vi "Device_without_barcode.vi"() -> ()   [LabVIEW 2016]
uses:
  Global_Valves.vi
  <vilib>/Utility/file.llb/Read Delimited Spreadsheet (I64).vi
panel:
  out "Plugs produced":dbl
  out "Elapsed time (min)":dbl
  out "Start time":timestamp
  out "Number of plugs":i64
  out "Duration of experiment (min)":dbl
  out "Horizontal Graduated Bar":u8(slide) max=66 scale=0.0..66.0
  out "Produced replicas":i32
  out "Inlets Flow On":bool[](array[boolean])
  out "Current condition":i32
  out "Current experiment iteration":i32
  in  "Abort":bool
  in  "Time-out Time":i32
  in  "Port":u16
  in  "Address":string
  out "Time Stamp":timestamp
  in  "Run experiment Button":bool
  out "Experiment running Led":bool
  in  "Experiment File":path
  out "Conditions with replica numbers":i64[][](array[numeric])
  out "Conditions array":i64[][](array[numeric])
  out "Replica numbers":i64[][](array[numeric])
  in  "Iterations of experiment":i32
  in  "Time of depressurization (ms)":u32
  in  "Time of pressurization (ms)":u32
  in  "Time of barcoding (ms)":u32
  in  "Inlet 9":bool
  in  "Inlet 10":bool
  in  "Inlet 11":bool
  in  "Inlet 12":bool
  in  "Inlet 13":bool
  in  "Inlet 14":bool
  in  "Inlet 15":bool
  in  "Inlet 16":bool
  out "Rows":i32
  out "Columns":i32
  in  "Pressurize all channels":bool
  in  "Depressurize all channels":bool
  in  "16":bool
  in  "15":bool
  in  "14":bool
  in  "13":bool
  in  "12":bool
  in  "11":bool
  in  "10":bool
  in  "9":bool
  in  "Stop button":bool
  # "Control \nChannels Manual Pressurization"
  # "Automatic Experiment"
  # "9"
  # "10"
  # "11"
  # "12"
  # "Barcode inlets"
  # "13"
  # "14"
  # "15"
  # "The Barcode Inlets buttons are not controlling anything\nYou can run the experiment without providing the barcode inlets.\n\nThe \"time of barcoding\" will be the time in between the different conditions, during which time all of the control channels are going to be pressurized and only oil will flow."
  # "16"
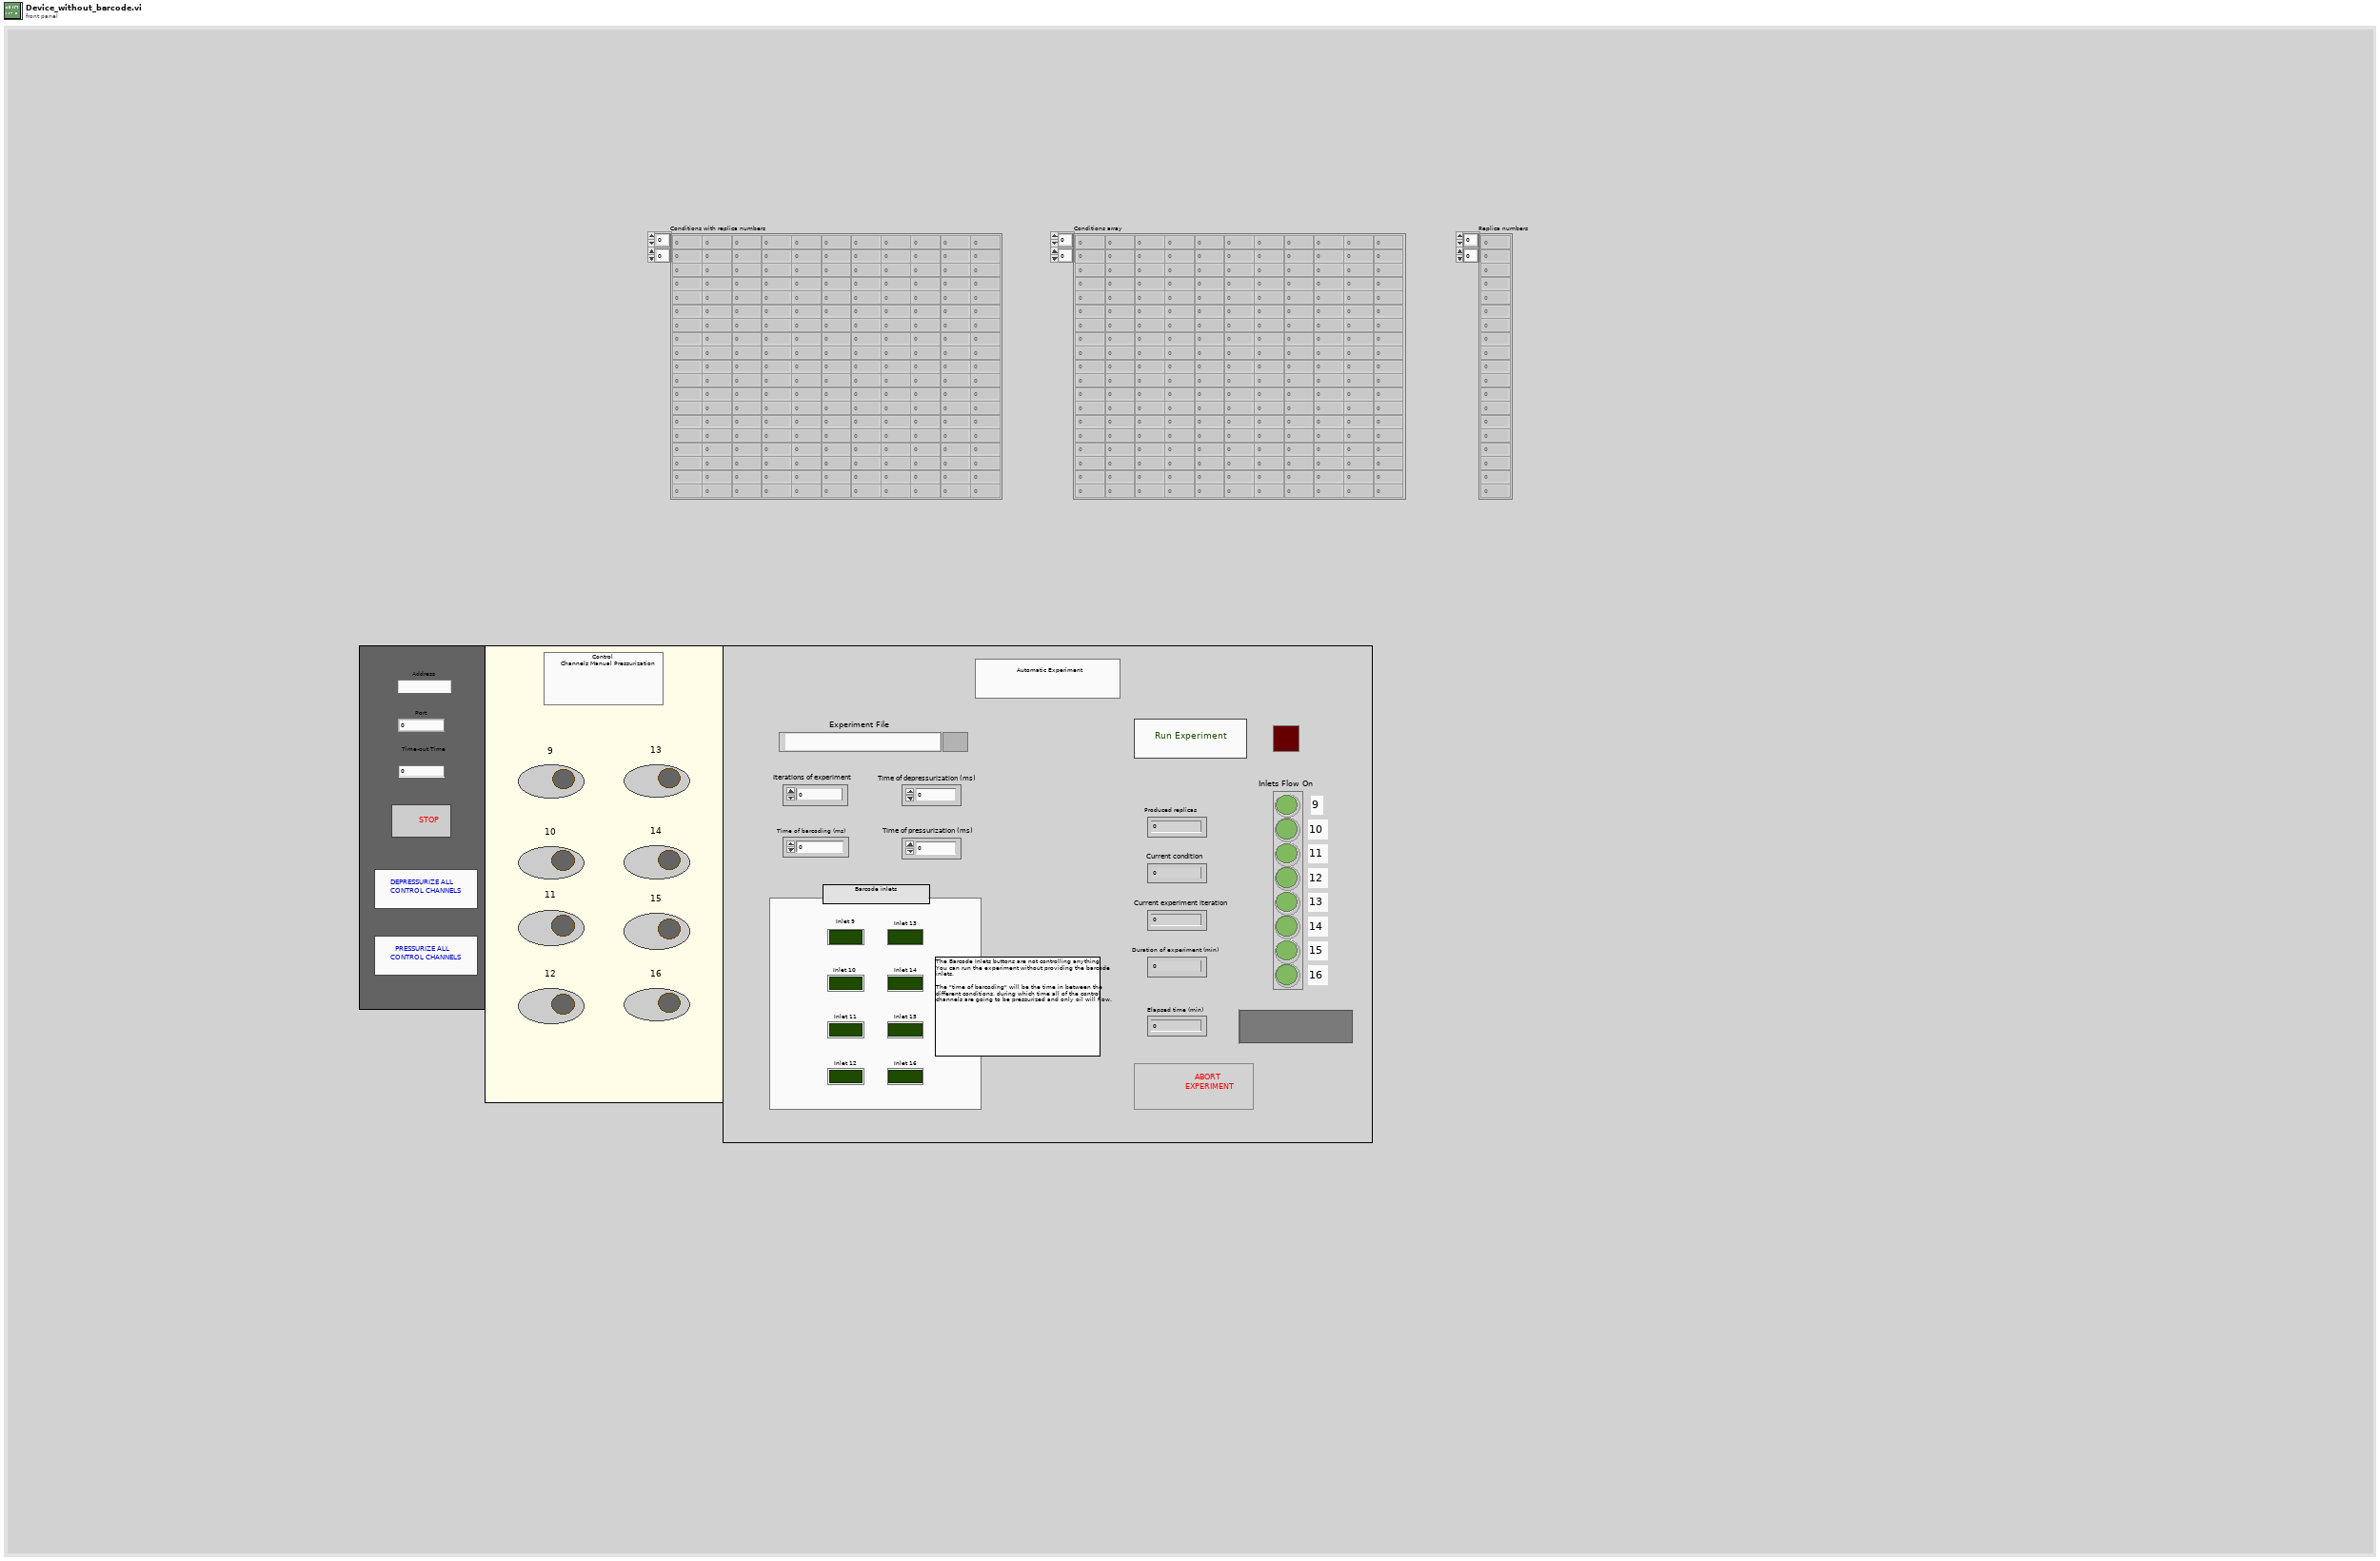
[diagram p1: front panel]
types:
  T1 = enum16{"Start", "Plug replicas production", "Barcoding", "Stop"}
  T2 = enum16{"Start", "Production of plug", "Close inlets", "Stop"}
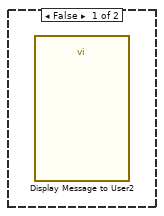
[diagram p2: hidden frame]
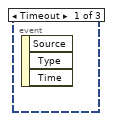
[diagram p4: hidden frame]
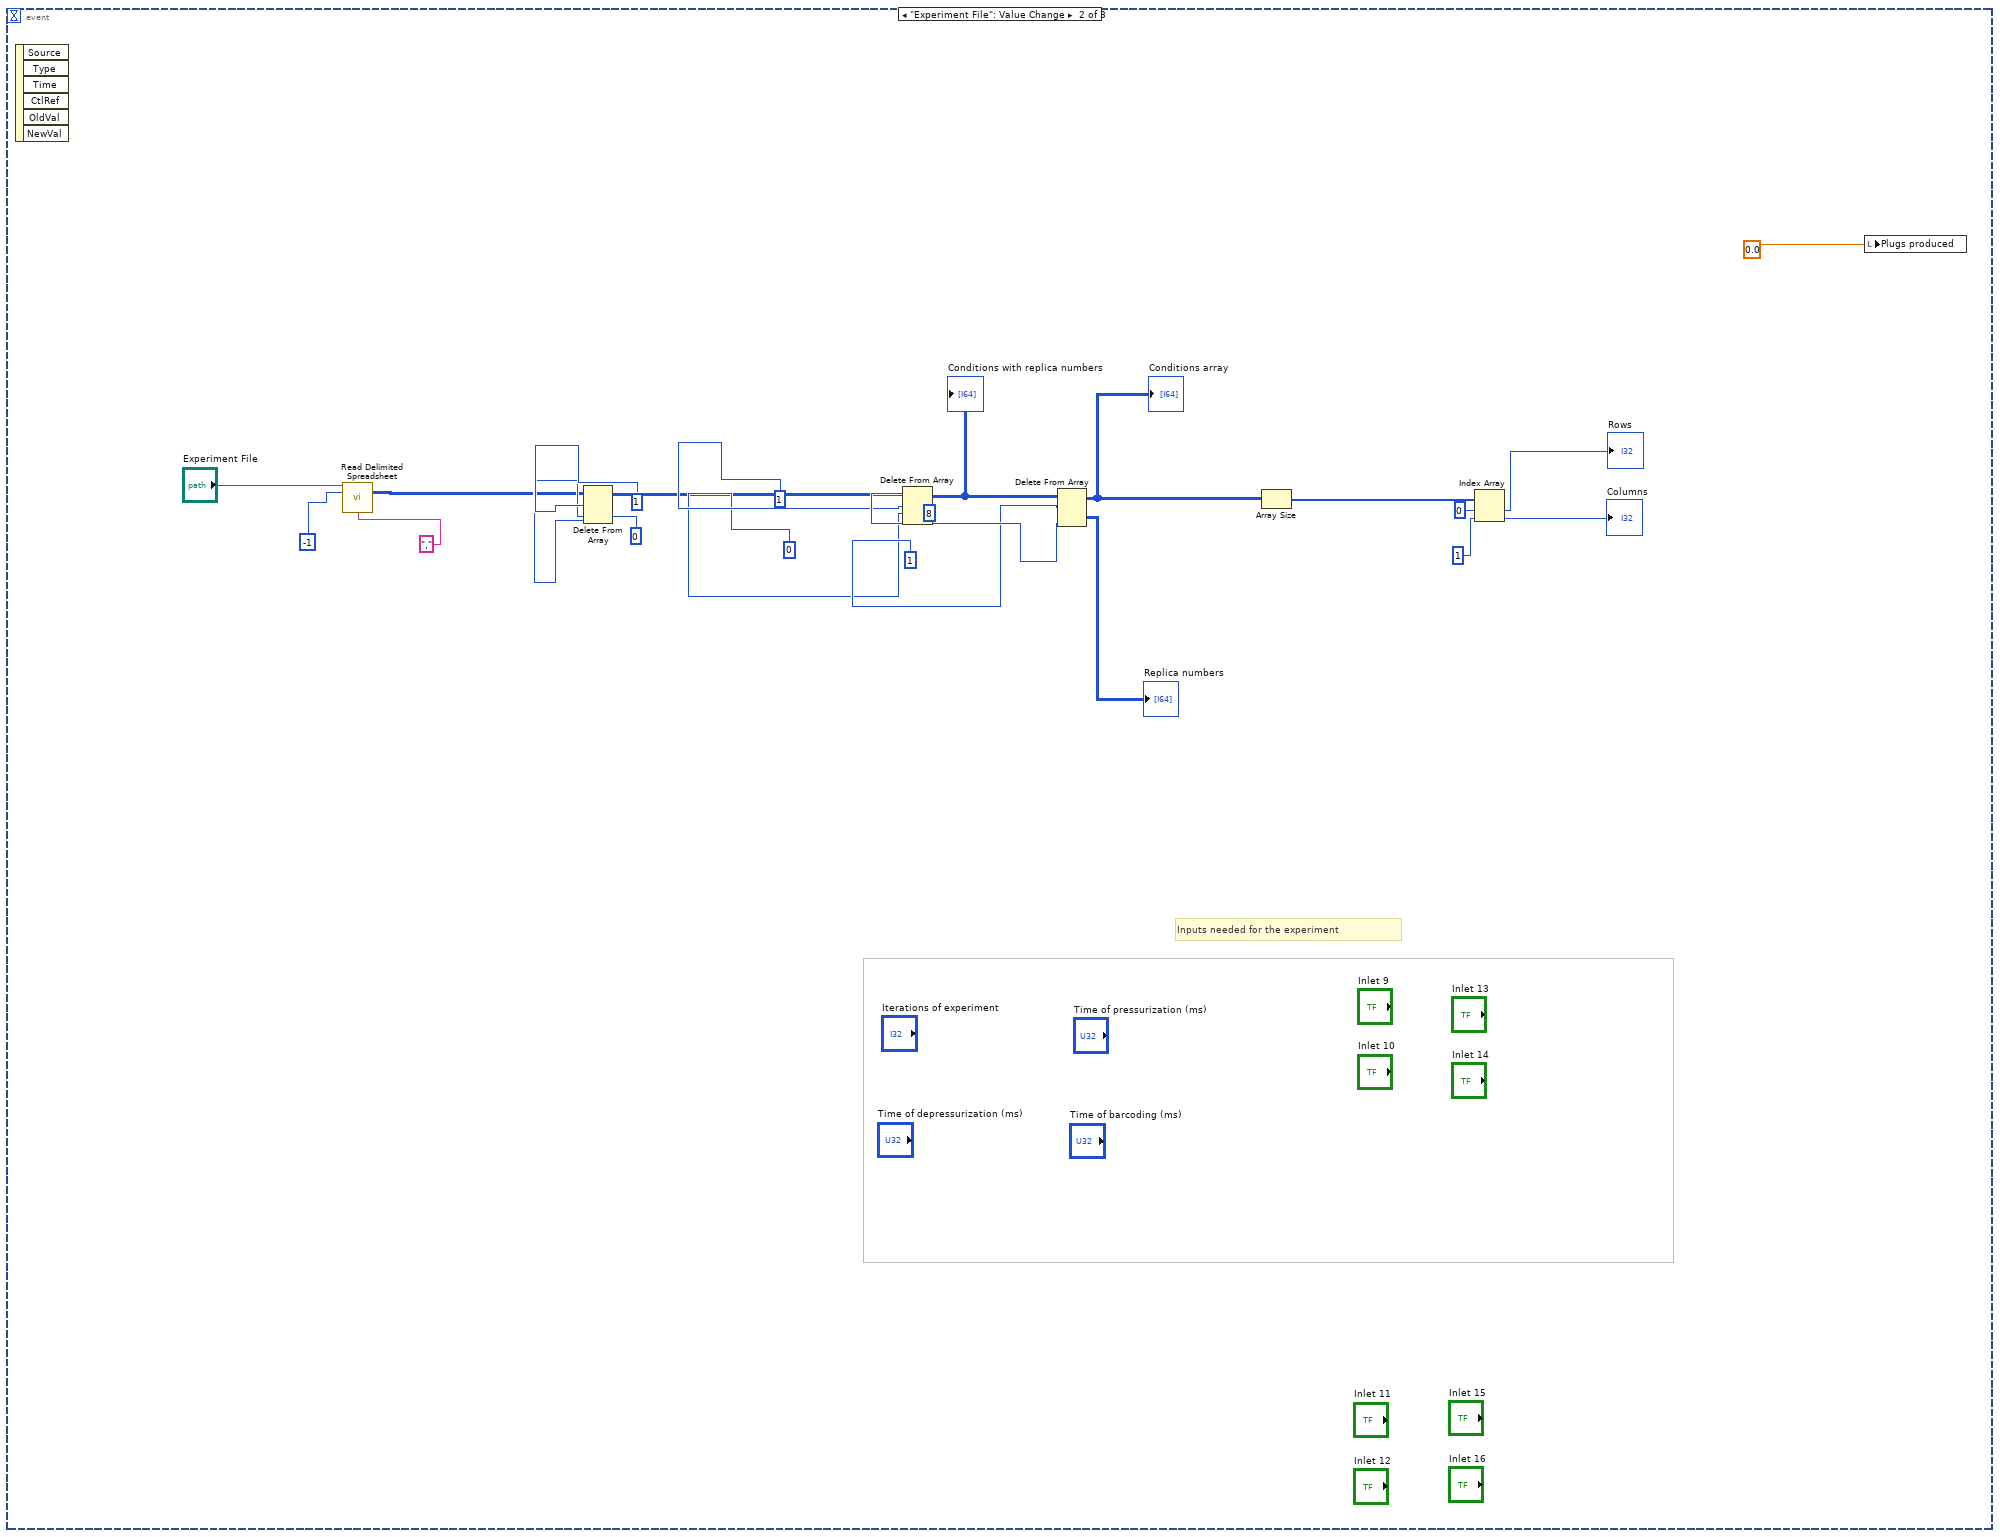
[diagram p5: hidden frame]
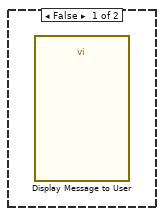
[diagram p6: hidden frame]
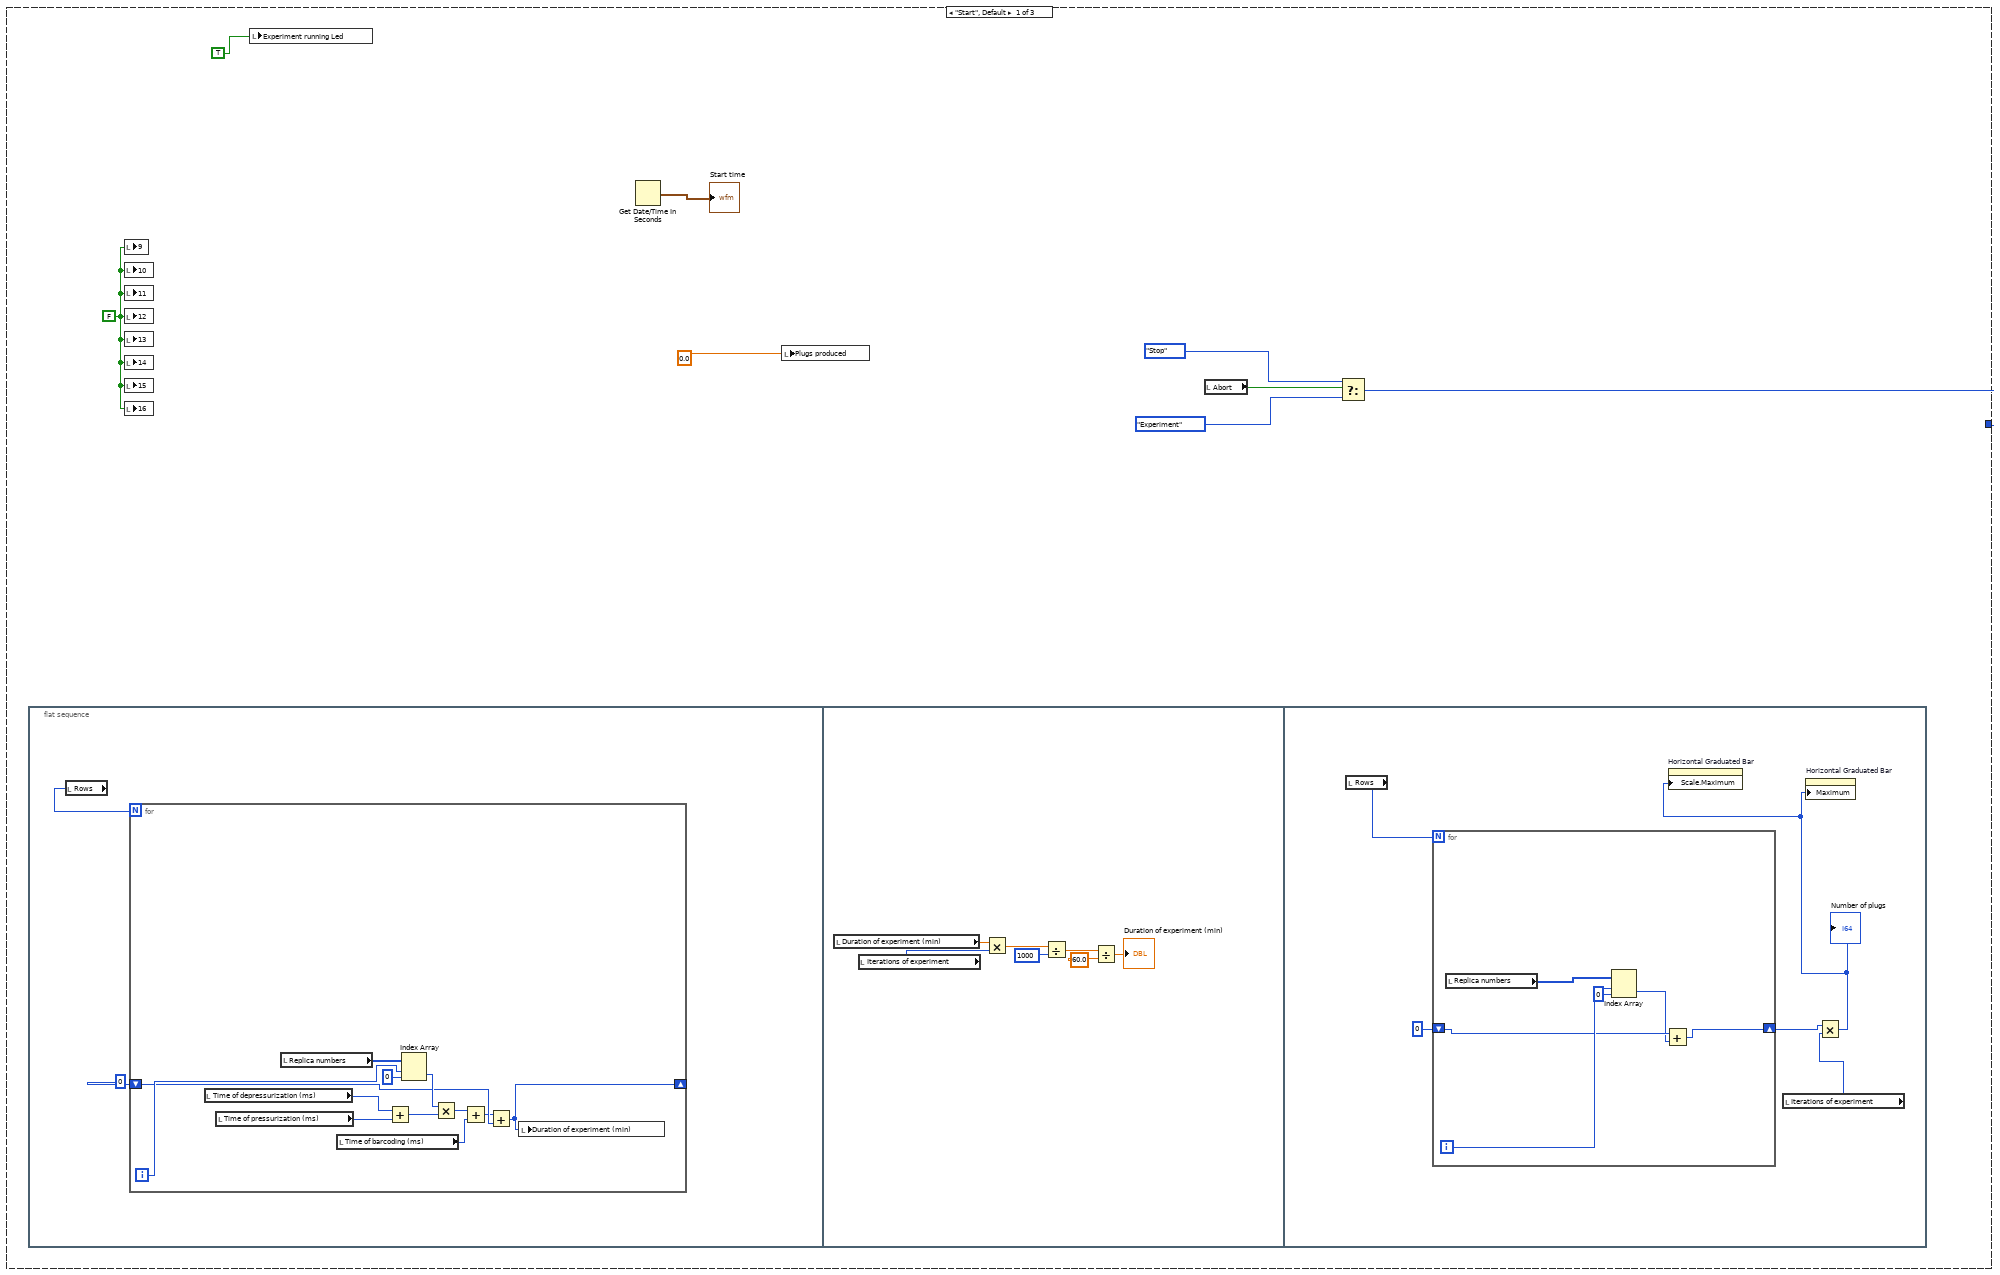
[diagram p7: hidden frame]
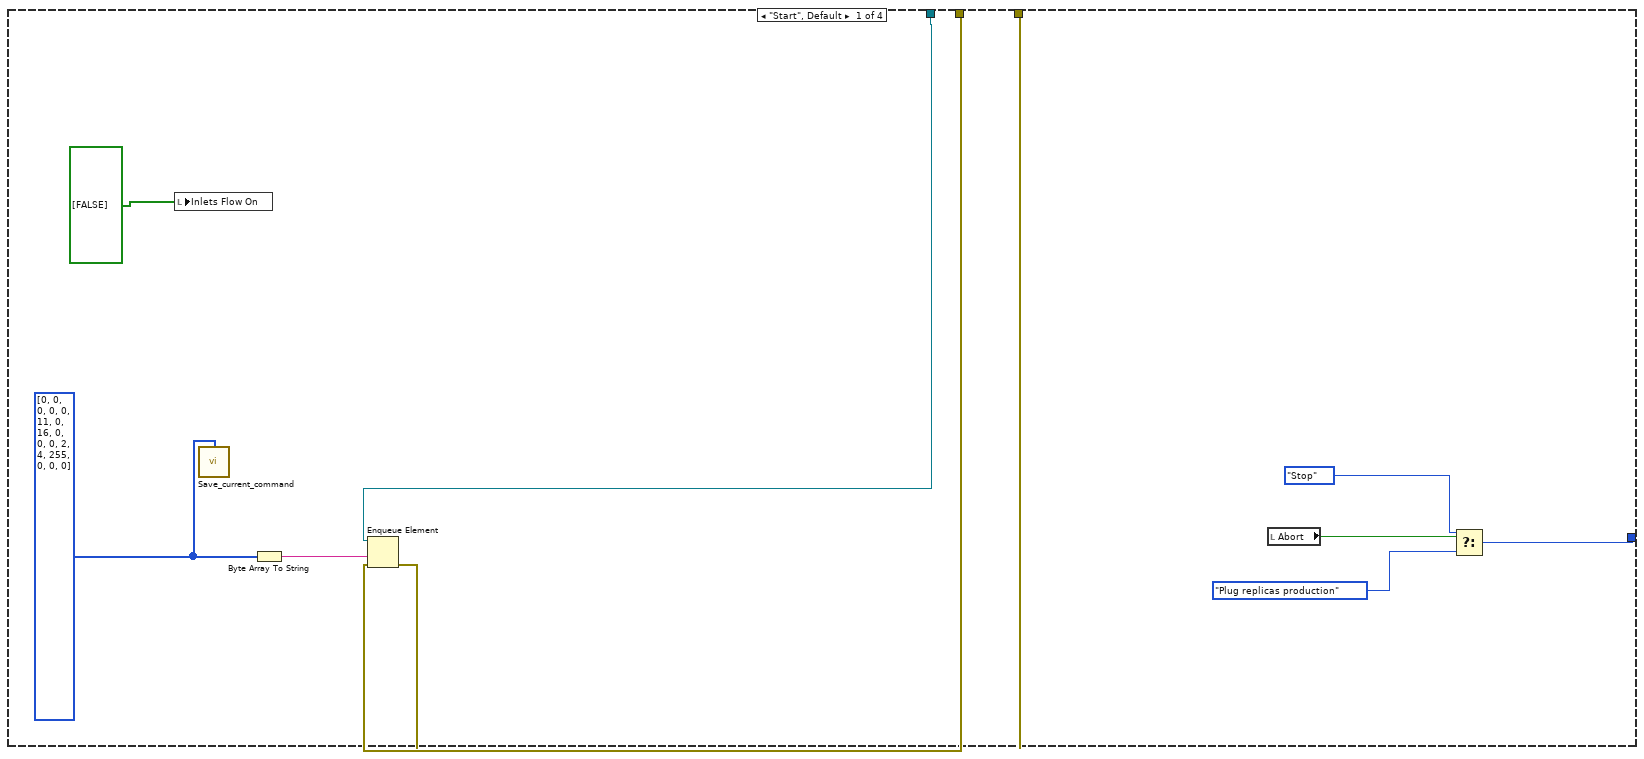
[diagram p8: hidden frame]
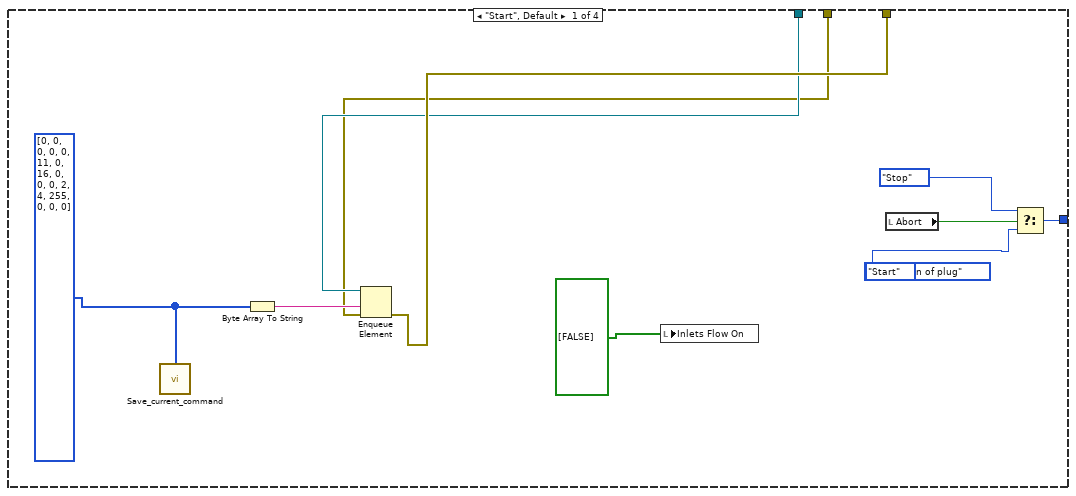
[diagram p9: hidden frame]
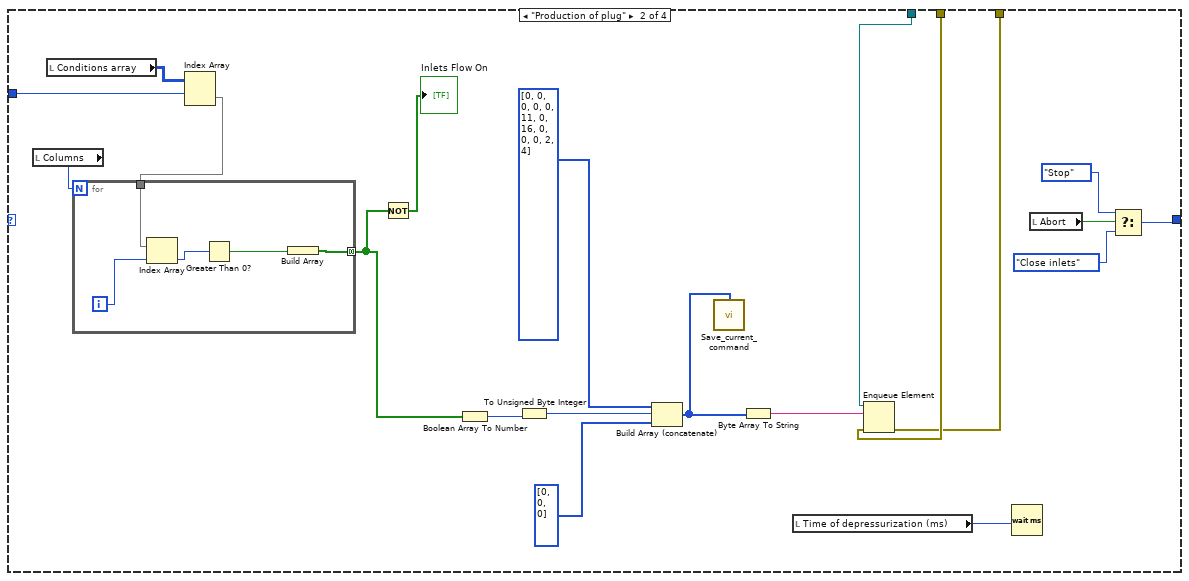
[diagram p10: hidden frame]
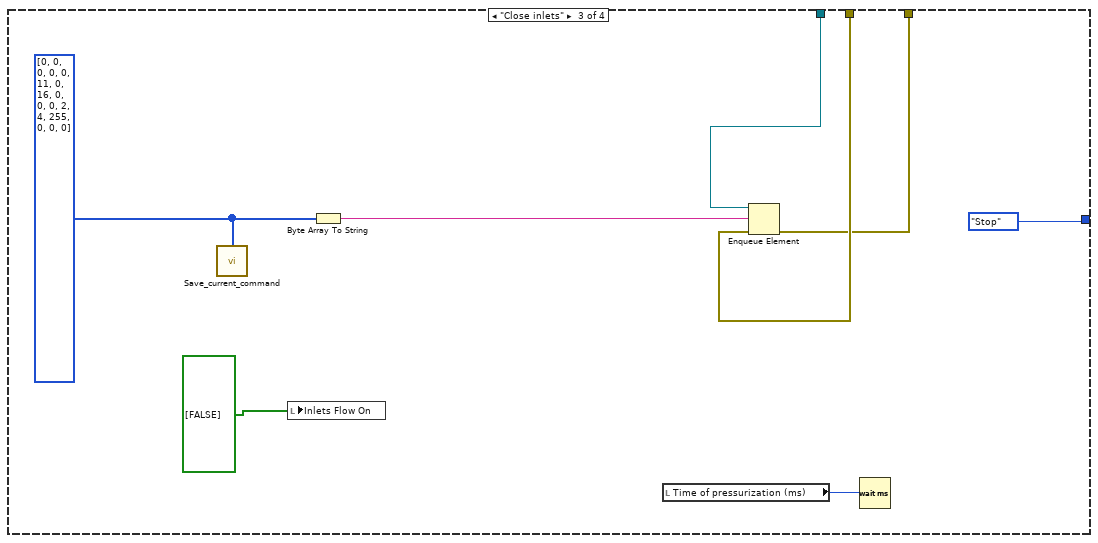
[diagram p11: hidden frame]
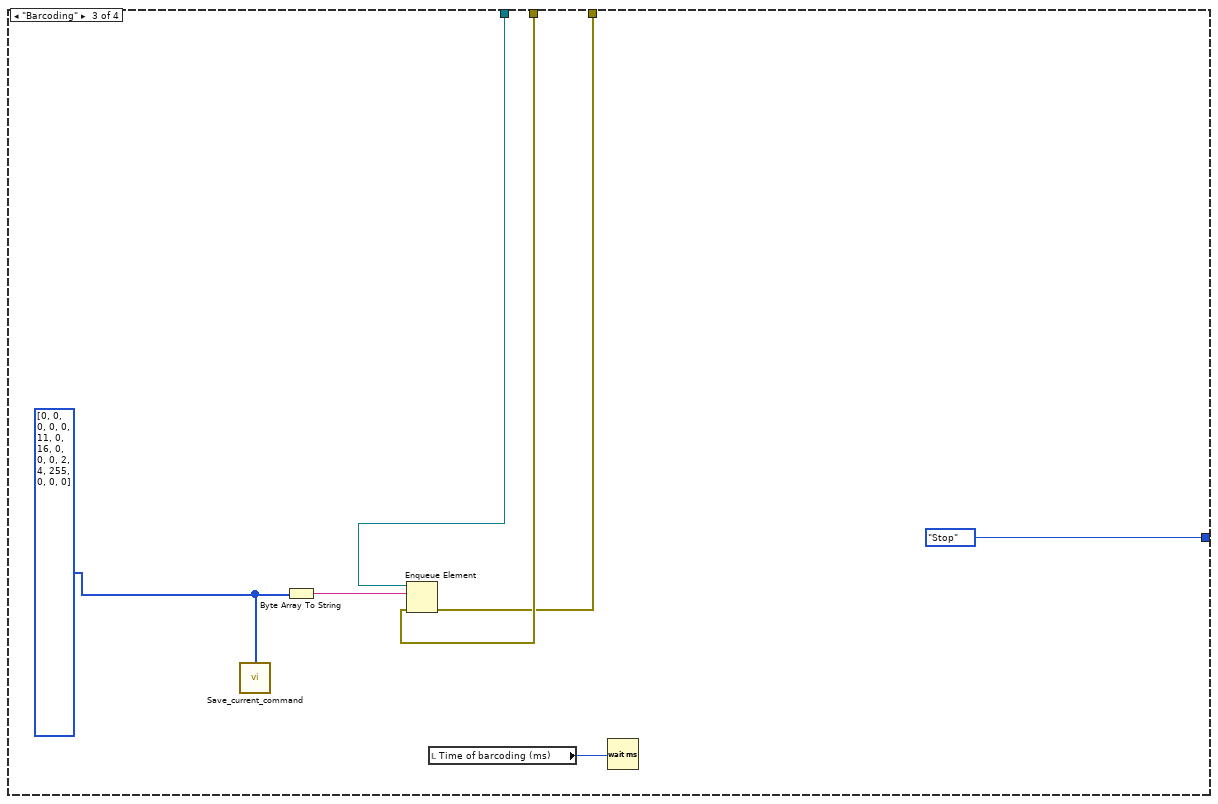
[diagram p12: hidden frame]
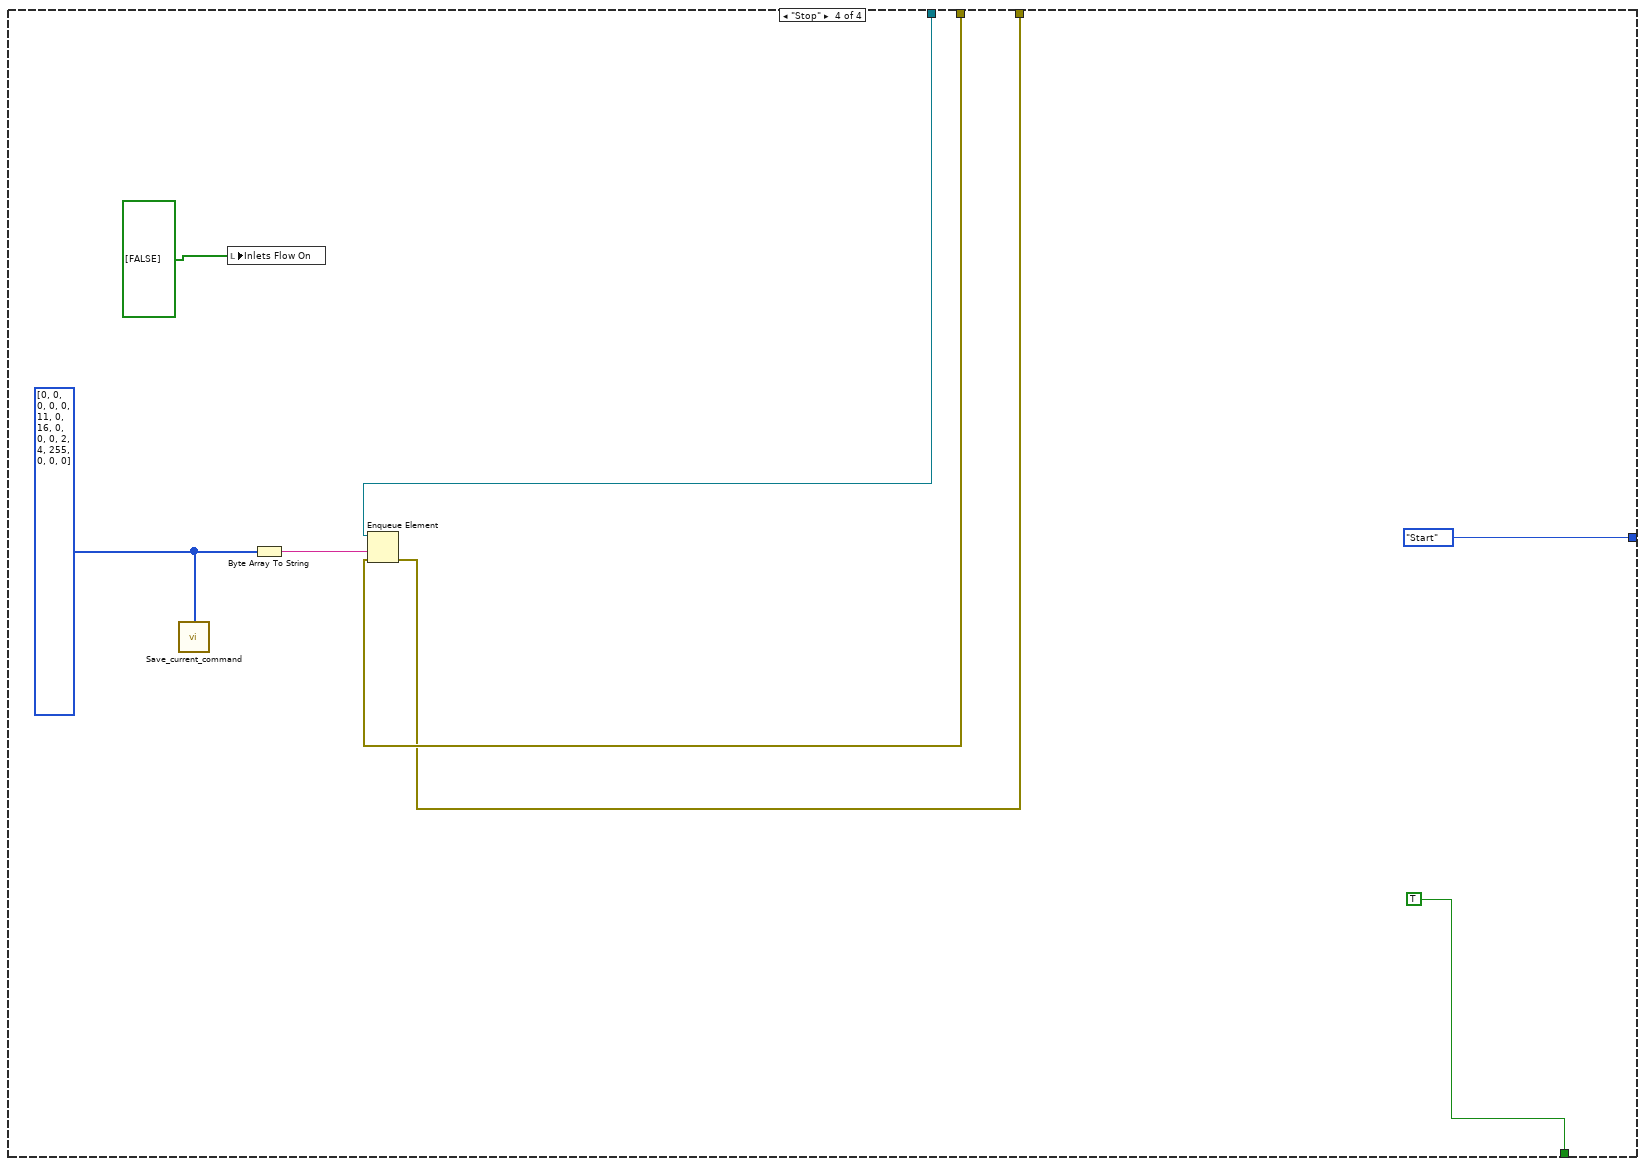
[diagram p13: hidden frame]
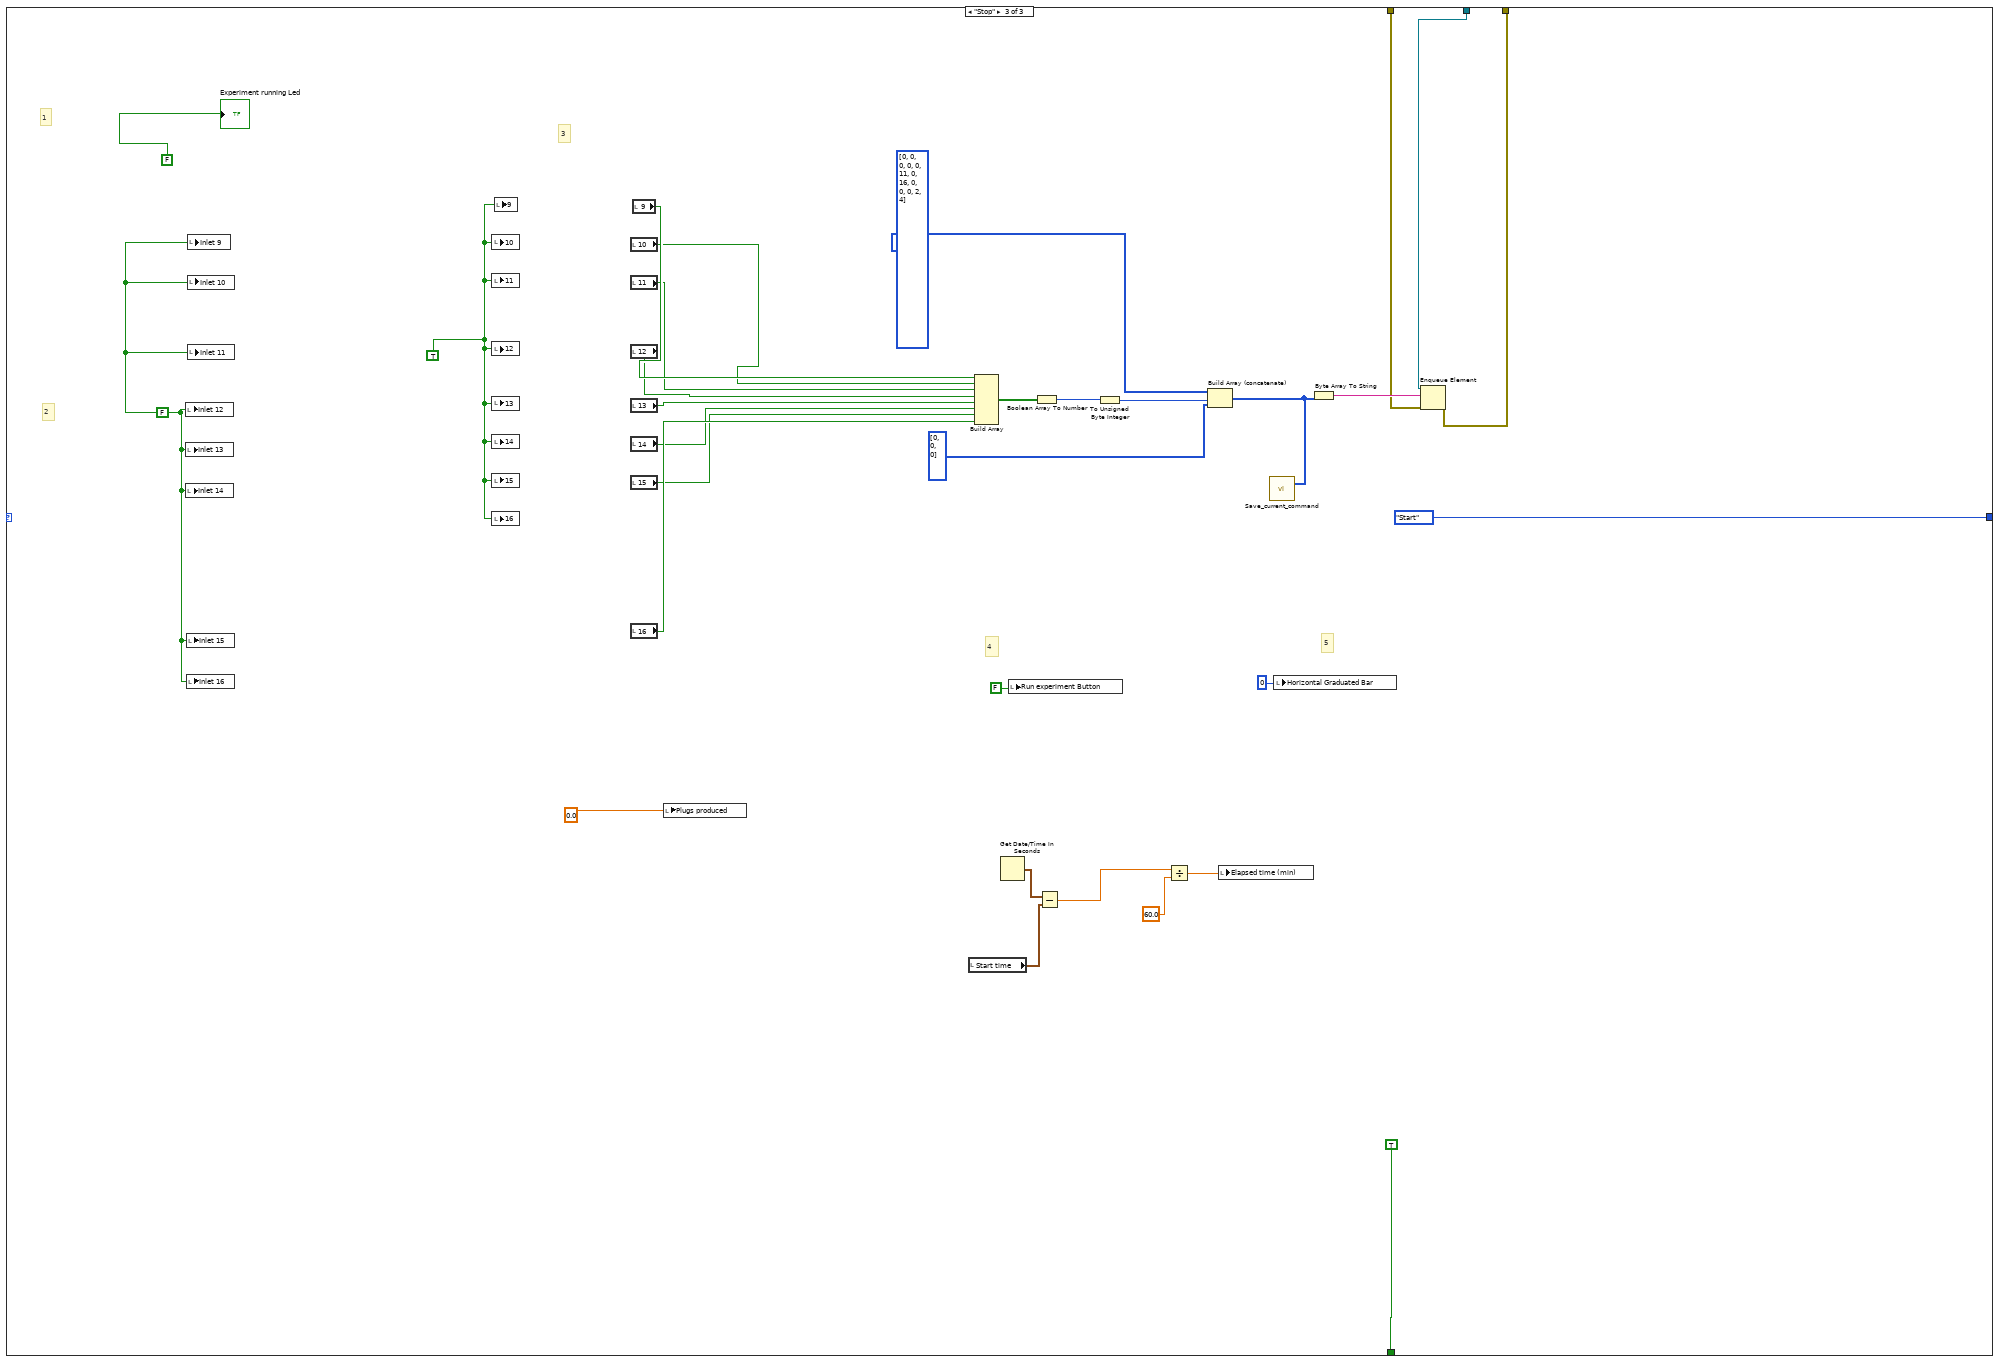
[diagram p14: hidden frame]
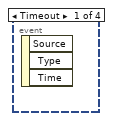
[diagram p15: hidden frame]
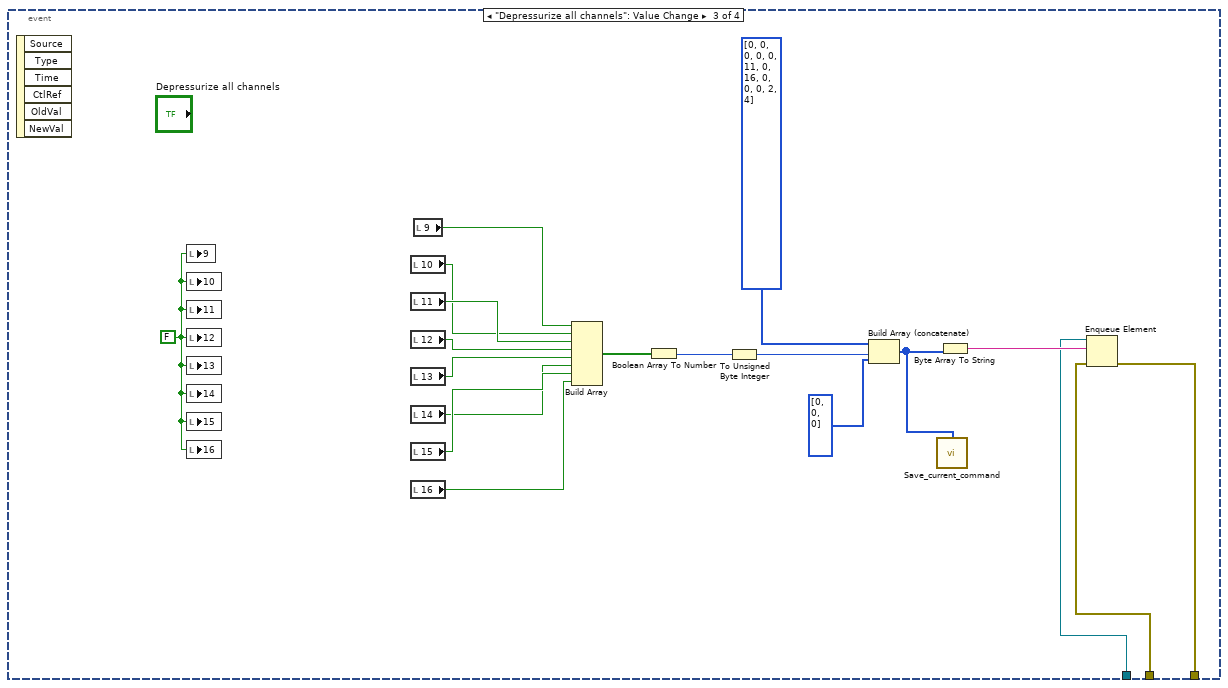
[diagram p16: hidden frame]
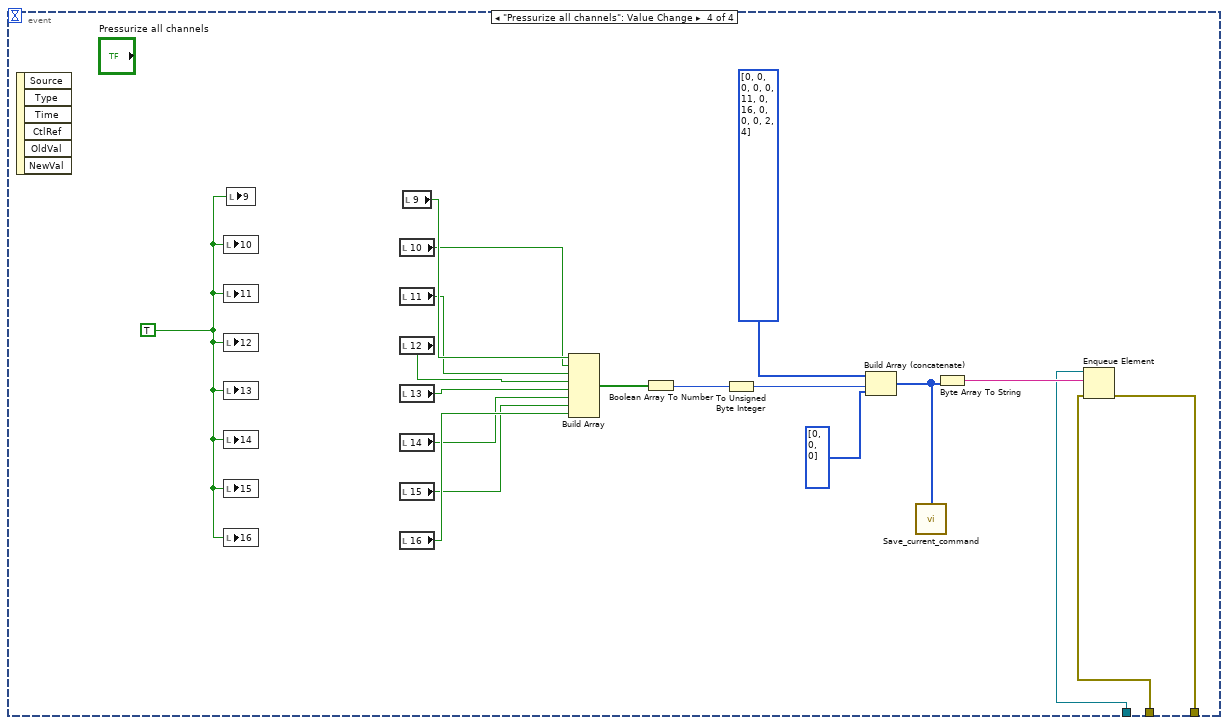
[diagram p17: hidden frame]
diagram:
  n1 = flat-sequence {
    frame #0 {
      # "2"
      # "1"
      # "FIRST SEQUENCE\n1. Checks if the user has provided the necessary tcp data\n2. Initialises the value of time stamp"
      n2 = String Length(string="Address") -> (length=w6:i32)
      n3 = Greater Than 0?(x=w6) -> (x > 0?=w5:bool)
      n4 = Greater Than 0?(x="Port") -> (x > 0?=w3:bool)
      n5 = Greater Than 0?(x="Time-out Time") -> (x > 0?=w1:bool)
      n6 = Get Date/Time In Seconds() -> (seconds since 1Jan1904=→"Time Stamp":timestamp)
      n7 = Compound Arithmetic op=AND(w5, w3, w1) -> (w8:bool)
      n8 = case shown="True" w8 {
        frame False {
          n9 = call "Display Message to User2"() -> ()  [unwired: 10 in, 2 out]
        }
        frame True {
        }
      }
    }
    frame #1 {
      w26 = "" ("name (unnamed)")
      # "WHILE LOOP B"
      # "WHILE LOOP C"
      # "3"
      # "WHILE LOOP E"
      # "WHILE LOOP D"
      # "WHILE LOOP A"
      # "SECOND 'SEQUENCE'\n1. ESTABLISH\n2. MAINTAIN TCP CONNECTION\n3. AUTOMATICALLY PRESSURIZE ALL CONTROLL CHANNELS -> FLOW PROHIBITED"
      # "2"
      # "1"
      n10 = Obtain Queue(name (unnamed)=w26, element data type=w26) -> (queue out=w12:refnum<queue>, error out=w11:errorcluster)  [unwired: 3 in, 1 out]
      n11 = while {
        tunnel: w12 -> [w32]
        tunnel: w11 -> [w31]
        tunnel: [w30] -> w10
        stop <- w29 stop-if-true
        n12 = local read "Time Stamp"() -> (w36:timestamp)
        n13 = Get Date/Time In Seconds() -> (seconds since 1Jan1904=w37:timestamp)
        n14 = Subtract(x=w37, y=w36) -> (x-y=w35:dbl)
        n15 = Greater?(x=w35, y=30.0) -> (0:w33:bool)
        n16 = case shown="True" w33 {
          tunnel: w32 -> [_ w55]
          tunnel: w31 -> [_ w49]
          tunnel: [_ w48] -> w30
          frame False {
          }
          frame True {
            n17 = global read "Global_Valves.vi" "Global valve 15"() -> (w41:bool)
            n18 = global read "Global_Valves.vi" "Global valve 16"() -> (w40:bool)
            n19 = global read "Global_Valves.vi" "Global valve 12"() -> (w44:bool)
            n20 = global read "Global_Valves.vi" "Global valve 11"() -> (w45:bool)
            n21 = global read "Global_Valves.vi" "Global valve 10"() -> (w46:bool)
            n22 = global read "Global_Valves.vi" "Global valve 13"() -> (w43:bool)
            n23 = global read "Global_Valves.vi" "Global valve 14"() -> (w42:bool)
            n24 = global read "Global_Valves.vi" "Global valve 9"() -> (w47:bool)
            n25 = Build Array(w47, w46, w45, w44, w43, w42, w41, w40) -> (w50:bool[])
            n26 = Get Date/Time In Seconds() -> (seconds since 1Jan1904=w56:timestamp)
            n27 = Boolean Array To Number(Boolean array=w50) -> (number=w51:u32)
            n28 = local write "Time Stamp"(w56) -> ()
            n29 = To Unsigned Byte Integer(number=w51) -> (unsigned 8bit integer=w53:u8)
            n30 = Build Array (concatenate)(u8[] [0, 0, 0, 0, 0, 11, 0, 16, 0, 0, 0, 2, 4] ("element"), w53, u8[] [0, 0, 0] ("element")) -> (w39:u8[])
            n31 = Byte Array To String(unsigned byte array=w39) -> (string=w38:string)
            n32 = Enqueue Element(queue=w55, element=w38, error in (no error)=w49) -> (error out=w48:errorcluster)  [unwired: 1 in, 2 out]
          }
        }
        n33 = local read "Stop button"() -> (w29:bool)
      }
      n34 = while {
        tunnel: w12 -> [w62]
        shift-right: [-1] -> _
        shift-left: 0 -> [w61]
        tunnel: w11 -> [w58]
        tunnel: [w57] -> w20
        stop <- w59 stop-if-true
        n35 = event shown="[0] Timeout" {
          selector: _ -> [_]
          dyn-events: _ -> [_]
          timeout: w61 -> [_]
          tunnel: w62 -> [w81]
          tunnel: w58 -> [w66]
          tunnel: [w65] -> w57
          event Timeout {
            w80 = TRUE
            n36 = event-data() -> ()  [unwired: 1 in, 3 out]
            n37 = local write "9"(w80) -> ()
            n38 = local write "10"(w80) -> ()
            n39 = local write "11"(w80) -> ()
            n40 = local write "12"(w80) -> ()
            n41 = local write "13"(w80) -> ()
            n42 = local write "14"(w80) -> ()
            n43 = local write "15"(w80) -> ()
            n44 = local write "16"(w80) -> ()
            n45 = local read "10"() -> (w69:bool)
            n46 = local read "11"() -> (w68:bool)
            n47 = local read "12"() -> (w67:bool)
            n48 = local read "13"() -> (w78:bool)
            n49 = local read "14"() -> (w77:bool)
            n50 = local read "15"() -> (w76:bool)
            n51 = local read "16"() -> (w75:bool)
            n52 = local read "9"() -> (w79:bool)
            n53 = Build Array(w79, w69, w68, w67, w78, w77, w76, w75) -> (w74:bool[])
            n54 = Boolean Array To Number(Boolean array=w74) -> (number=w73:u32)
            n55 = To Unsigned Byte Integer(number=w73) -> (unsigned 8bit integer=w70:u8)
            n56 = Build Array (concatenate)(u8[] [0, 0, 0, 0, 0, 11, 0, 16, 0, 0, 0, 2, 4] ("element"), w70, u8[] [0, 0, 0] ("element")) -> (w63:u8[])
            n57 = call "Save_current_command.vi"("Array"=w63) -> ()  [unwired: 15 in]
            n58 = Byte Array To String(unsigned byte array=w63) -> (string=w71:string)
            n59 = Enqueue Element(queue=w81, element=w71, error in (no error)=w66) -> (error out=w65:errorcluster)  [unwired: 1 in, 2 out]
          }
        }
        n60 = First Call?() -> (First Call?: T/F=w59:bool)
      }
      n61 = local read "Time-out Time"() -> (w16:i32)
      n62 = local read "Address"() -> (w18:string)
      n63 = local read "Port"() -> (w17:u16)
      n64 = TCP Open Connection(address=w18, remote port or service name=w17, timeout ms (60000)=w16) -> (connection ID=w22:refnum<k5>, error out=w23:errorcluster)  [unwired: 2 in]
      n65 = while {
        tunnel: w22 -> [w348]
        tunnel: w23 -> [w347]
        tunnel: [w346] -> w24
        tunnel: [w345] -> w25
        tunnel: w12 -> [w344]
        tunnel: w11 -> [w343]
        tunnel: [w341] -> w21
        tunnel: [w339] -> w15
        stop <- w340 stop-if-true
        n66 = Dequeue Element(queue=w344, error in (no error)=w343) -> (queue out=w339:refnum<queue>, element=w342:string, error out=w341:errorcluster)  [unwired: 1 in, 1 out]
        n67 = call "TCP_WRITE_READ_SV.vi"("error in (no error)"=w347, "command"=w342, "TCP Network Connection in"=w348) -> ("error out"=w345:errorcluster, "TCP Network Connection out"=w346:refnum<k5>)  [unwired: 7 in]
        n68 = local read "Stop button"() -> (w340:bool)
      }
      n69 = TCP Close Connection(connection ID=w24, error in (no error)=w25) -> (error out=w28:errorcluster)  [unwired: 1 in, 1 out]
      n70 = call <vilib>:"Simple Error Handler.vi"("error in (no error)"=w28) -> ()  [unwired: 4 in, 5 out]
      n71 = while {
        tunnel: w12 -> [w84]
        tunnel: w11 -> [w83]
        tunnel: [w82] -> w14
        stop <- w85 stop-if-true
        n72 = event shown="[2] \"Run experiment Button\": Value Change" {
          selector: _ -> [_ _ _]
          dyn-events: _ -> [_ _ _]
          timeout: _ -> [_ _ _]
          tunnel: w84 -> [_ _ w109]
          tunnel: w83 -> [_ _ w108]
          tunnel: [_ _ w107] -> w82
          event Timeout {
            n73 = event-data() -> ()  [unwired: 1 in, 3 out]
          }
          event "Experiment File": Value Change {
            # "Inputs needed for the experiment"
            n74 = event-data() -> ()  [unwired: 1 in, 6 out]
            n75 = call-poly <vilib>:"Read Delimited Spreadsheet.vi"("file path (dialog if empty)"="Experiment File", "number of rows (all:-1)"=-1, "delimiter (\\t)"="," ("delimiter (\\t)")) -> ("all rows"=w90:i64[][])  [unwired: 7 in, 5 out]
            n76 = Delete From Array(array=w90, length=1, index (col)=0 ("disabled index (col)")) -> (array with subset deleted=w96:i64[][])  [unwired: 1 in, 1 out]
            n77 = Delete From Array(array=w96, length=1, index (row)=0) -> (array with subset deleted=w99:i64[][])  [unwired: 1 in, 1 out]
            "Conditions with replica numbers" <- w99
            n78 = Delete From Array(array=w99, length=1, index (col)=8 ("disabled index (col)")) -> (deleted portion=→"Replica numbers":i64[][], array with subset deleted=w102:i64[][])  [unwired: 1 in]
            "Conditions array" <- w102
            n79 = Array Size(array=w102) -> (size(s)=w89:i32[])
            n80 = Index Array(array=w89, index #1=0 ("index"), index #2=1 ("index")) -> (element #1=→"Rows":i32, element #2=→"Columns":i32)
            n81 = local write "Plugs produced"(0.0 ("plugs")) -> ()
          }
          event "Run experiment Button": Value Change {
            n82 = event-data() -> ()  [unwired: 1 in, 6 out]
            n83 = local read "Time of depressurization (ms)"() -> (w116:u32)
            n84 = local read "Time of pressurization (ms)"() -> (w118:u32)
            n85 = local read "Time of barcoding (ms)"() -> (w119:u32)
            n86 = local read "Iterations of experiment"() -> (w117:i32)
            n87 = Greater Than 0?(x=w119) -> (x > 0?=w115:bool)
            n88 = Greater Than 0?(x=w118) -> (x > 0?=w114:bool)
            n89 = Greater Than 0?(x=w116) -> (x > 0?=w112:bool)
            n90 = Greater Than 0?(x=w117) -> (x > 0?=w113:bool)
            n91 = And(x=w115, y=w114) -> (x .and. y?=w111:bool)
            n92 = And(x=w113, y=w112) -> (x .and. y?=w110:bool)
            n93 = And(x=w111, y=w110) -> (x .and. y?=w106:bool)
            n94 = case shown="True" w106 {
              tunnel: w109 -> [_ w122]
              tunnel: w108 -> [_ w121]
              tunnel: [_ w120] -> w107
              frame False {
                n95 = call "Display Message to User"() -> ()  [unwired: 10 in, 2 out]
              }
              frame True {
                n96 = while {
                  shift-right: [w128] -> _
                  shift-left: enum16{"Start", "Experiment", "Stop"}."Start" -> [w129]
                  tunnel: w122 -> [w126]
                  tunnel: w121 -> [w125]
                  tunnel: [w124] -> w120
                  stop <- w127 stop-if-true
                  n97 = case shown="\"Experiment\"" w129 {
                    tunnel: [w133 enum16{"Start", "Experiment", "Stop"}."Stop" enum16{"Start", "Experiment", "Stop"}."Start"] -> w128
                    tunnel: [_ _ TRUE] -> w127
                    tunnel: w126 -> [_ w172 w319]
                    tunnel: w125 -> [_ w171 w318]
                    tunnel: [_ w170 w317] -> w124
                    frame "Start", Default {
                      w137 = FALSE
                      n98 = flat-sequence {
                        frame #0 {
                          n99 = local read "Rows"() -> (w139:i32)
                          n100 = for {
                            N: w139 -> [_]
                            shift-right: [w140] -> _
                            shift-left: 0 -> [w143]
                            i -> [w150]
                            n101 = local read "Time of depressurization (ms)"() -> (w147:u32)
                            n102 = local read "Time of pressurization (ms)"() -> (w148:u32)
                            n103 = local read "Replica numbers"() -> (w151:i64[][])
                            n104 = local read "Time of barcoding (ms)"() -> (w144:u32)
                            n105 = Add(x=w147, y=w148) -> (x+y=w149:u32)
                            n106 = Index Array(array=w151, index (row)=w150, index (col)=0 ("disabled index (col)")) -> (element=w146:i64)
                            n107 = Multiply(x=w146, y=w149) -> (x*y=w145:i64)
                            n108 = Add(x=w145, y=w144) -> (x+y=w142:i64)
                            n109 = Add(x=w142, y=w143) -> (x+y=w140:i64)
                            n110 = local write "Duration of experiment (min)"(w140) -> ()
                          }
                        }
                        frame #1 {
                          n111 = local read "Duration of experiment (min)"() -> (w155:dbl)
                          n112 = local read "Iterations of experiment"() -> (w158:i32)
                          n113 = Multiply(x=w155, y=w158) -> (x*y=w157:dbl)
                          n114 = Divide(x=w157, y=i64 1000) -> (x/y=w154:dbl)
                          n115 = Divide(x=w154, y=60.0) -> (x/y=→"Duration of experiment (min)":dbl)
                        }
                        frame #2 {
                          n116 = local read "Rows"() -> (w163:i32)
                          n117 = for {
                            N: w163 -> [_]
                            shift-right: [w164] -> w161
                            shift-left: i64 0 ("Replica numbers") -> [w166]
                            i -> [w168]
                            n118 = local read "Replica numbers"() -> (w169:i64[][])
                            n119 = Index Array(array=w169, index (row)=w168, index (col)=0 ("disabled index (col)")) -> (element=w165:i64)
                            n120 = Add(x=w166, y=w165) -> (x+y=w164:i64)
                          }
                          n121 = local read "Iterations of experiment"() -> (w160:i32)
                          n122 = Multiply(x=w161, y=w160) -> (x*y=w159:i64)
                          "Number of plugs" <- w159
                          n123 = property on="Horizontal Graduated Bar" class="Slide (strict)"("Scale.Maximum"=w159) -> ()  [unwired: 2 in, 2 out]
                          n124 = property on="Horizontal Graduated Bar" class="Slide (strict)"("Maximum"=w159) -> ()  [unwired: 2 in, 2 out]
                        }
                      }
                      n125 = local write "9"(w137) -> ()
                      n126 = local write "10"(w137) -> ()
                      n127 = local write "11"(w137) -> ()
                      n128 = local write "12"(w137) -> ()
                      n129 = local write "13"(w137) -> ()
                      n130 = local write "14"(w137) -> ()
                      n131 = local write "15"(w137) -> ()
                      n132 = local write "16"(w137) -> ()
                      n133 = local write "Experiment running Led"(TRUE ("Boolean")) -> ()
                      n134 = Get Date/Time In Seconds() -> (seconds since 1Jan1904=→"Start time":timestamp)
                      n135 = local write "Plugs produced"(0.0 ("plugs")) -> ()
                      n136 = local read "Abort"() -> (w135:bool)
                      n137 = Select(t=enum16{"Start", "Experiment", "Stop"}."Stop", s=w135, f=enum16{"Start", "Experiment", "Stop"}."Experiment") -> (s? t:f=w133:enum16{"Start", "Experiment", "Stop"})
                    }
                    frame "Experiment" {
                      n138 = local read "Iterations of experiment"() -> (w174:i32)
                      n139 = for {
                        N: w174 -> [_]
                        tunnel: w172 -> [w178]
                        tunnel: w171 -> [w177]
                        tunnel: [w176] -> w170
                        i -> [w180]
                        stop <- "Abort" stop-if-true
                        n140 = local read "Rows"() -> (w175:i32)
                        n141 = Increment(x=w180) -> (x+1=→"Current experiment iteration":i32)
                        n142 = for {
                          N: w175 -> [_]
                          tunnel: w178 -> [w185]
                          tunnel: w177 -> [w184]
                          tunnel: [w183] -> w176
                          i -> [w186]
                          stop <- w189 stop-if-true
                          n143 = local read "Replica numbers"() -> (w190:i64[][])
                          n144 = Increment(x=w186) -> (x+1=→"Current condition":i32)
                          n145 = Index Array(array=w190, index (row)=w186, index (col)=0) -> (element=w188:i64)
                          n146 = while {
                            shift-right: [w199] -> _
                            shift-left: T1."Start" -> [w196]
                            tunnel: w188 -> [w197]
                            tunnel: w186 -> [w195]
                            tunnel: w185 -> [w193]
                            tunnel: w184 -> [w192]
                            tunnel: [w194] -> w183
                            stop <- w198 stop-if-true
                            n147 = case shown="\"Plug replicas production\"" w196 {
                              tunnel: [w207 w218 T1."Stop" T1."Start"] -> w199
                              tunnel: [_ _ _ TRUE] -> w198
                              tunnel: w197 -> [_ w210 _ _]
                              tunnel: w195 -> [_ w214 _ _]
                              tunnel: w193 -> [w204 w213 w296 w303]
                              tunnel: w192 -> [w203 w212 w295 w302]
                              tunnel: [w202 w211 w294 w301] -> w194
                              frame "Start", Default {
                                w200 = u8[] [0, 0, 0, 0, 0, 11, 0, 16, 0, 0, 0, 2, 4, 255, 0, 0, 0] ("element")
                                n148 = local write "Inlets Flow On"(bool[] [FALSE] ("Inlets On")) -> ()
                                n149 = call "Save_current_command.vi"("Array"=w200) -> ()  [unwired: 15 in]
                                n150 = Byte Array To String(unsigned byte array=w200) -> (string=w206:string)
                                n151 = Enqueue Element(queue=w204, element=w206, error in (no error)=w203) -> (error out=w202:errorcluster)  [unwired: 1 in, 2 out]
                                n152 = local read "Abort"() -> (w209:bool)
                                n153 = Select(t=T1."Stop", s=w209, f=T1."Plug replicas production") -> (s? t:f=w207:T1)
                              }
                              frame "Plug replicas production" {
                                n154 = for {
                                N: w210 -> [_]
                                tunnel: w214 -> [w226]
                                tunnel: w213 -> [w224]
                                tunnel: w212 -> [w223]
                                tunnel: [w225] -> w211
                                tunnel: w210 -> [_]
                                shift-right: [w219] -> _
                                shift-left: _ -> [w220]
                                i -> [w222]
                                stop <- w228 stop-if-true
                                n155 = Increment(x=w222) -> (x+1=→"Produced replicas":i32)
                                n156 = while {
                                shift-right: [w234] -> _
                                shift-left: T2."Start" -> [w236]
                                tunnel: w226 -> [w233]
                                tunnel: w224 -> [w232]
                                tunnel: w223 -> [w231]
                                tunnel: [w230] -> w225
                                i -> [w229]
                                stop <- w235 stop-if-true
                                n157 = case shown="\"Stop\"" w236 {
                                tunnel: [_ _ _ TRUE] -> w235
                                tunnel: [w246 w266 T2."Stop" T2."Start"] -> w234
                                tunnel: w233 -> [_ w255 _ _]
                                tunnel: w232 -> [w239 w251 w275 w288]
                                tunnel: w231 -> [w238 w250 w274 w287]
                                tunnel: [w241 w249 w273 w286] -> w230
                                tunnel: w229 -> [_ _ _ _]
                                frame "Start", Default {
                                w237 = u8[] [0, 0, 0, 0, 0, 11, 0, 16, 0, 0, 0, 2, 4, 255, 0, 0, 0] ("element")
                                (unwired) T2."Start"
                                n158 = call "Save_current_command.vi"("Array"=w237) -> ()  [unwired: 15 in]
                                n159 = Byte Array To String(unsigned byte array=w237) -> (string=w242:string)
                                n160 = Enqueue Element(queue=w239, element=w242, error in (no error)=w238) -> (error out=w241:errorcluster)  [unwired: 1 in, 2 out]
                                n161 = local write "Inlets Flow On"(bool[] [FALSE] ("Inlets On")) -> ()
                                n162 = local read "Abort"() -> (w245:bool)
                                n163 = Select(t=T2."Stop", s=w245, f=T2."Production of plug") -> (s? t:f=w246:T2)
                                }
                                frame "Production of plug" {
                                n164 = local read "Columns"() -> (w257:i32)
                                n165 = local read "Conditions array"() -> (w256:i64[][])
                                n166 = Index Array(array=w256, index (row)=w255) -> (element=w254:i64[])  [unwired: 1 in]
                                n167 = for {
                                N: w257 -> [_]
                                tunnel: w254 -> [w271]
                                tunnel: [w267] -> w248 mode=concatenating
                                i -> [w270]
                                n168 = Index Array(array=w271, index=w270) -> (element=w269:i64)
                                n169 = Greater Than 0?(x=w269) -> (x > 0?=w268:bool)
                                n170 = Build Array(w268) -> (w267:bool[])
                                }
                                n171 = Not(x=w248) -> (.not. x?=→"Inlets Flow On":bool[])
                                n172 = Boolean Array To Number(Boolean array=w248) -> (number=w253:u32)
                                n173 = To Unsigned Byte Integer(number=w253) -> (unsigned 8bit integer=w259:u8)
                                n174 = Build Array (concatenate)(u8[] [0, 0, 0, 0, 0, 11, 0, 16, 0, 0, 0, 2, 4] ("element"), w259, u8[] [0, 0, 0] ("element")) -> (w247:u8[])
                                n175 = call "Save_current_command.vi"("Array"=w247) -> ()  [unwired: 15 in]
                                n176 = Byte Array To String(unsigned byte array=w247) -> (string=w262:string)
                                n177 = local read "Time of depressurization (ms)"() -> (w258:u32)
                                n178 = Enqueue Element(queue=w251, element=w262, error in (no error)=w250) -> (error out=w249:errorcluster)  [unwired: 1 in, 2 out]
                                n179 = Wait (ms)(milliseconds to wait=w258) -> ()  [unwired: 1 out]
                                n180 = local read "Abort"() -> (w265:bool)
                                n181 = Select(t=T2."Stop", s=w265, f=T2."Close inlets") -> (s? t:f=w266:T2)
                                }
                                frame "Close inlets" {
                                w272 = u8[] [0, 0, 0, 0, 0, 11, 0, 16, 0, 0, 0, 2, 4, 255, 0, 0, 0] ("element")
                                n182 = call "Save_current_command.vi"("Array"=w272) -> ()  [unwired: 15 in]
                                n183 = local write "Inlets Flow On"(bool[] [FALSE] ("Inlets On")) -> ()
                                n184 = Byte Array To String(unsigned byte array=w272) -> (string=w276:string)
                                n185 = local read "Time of pressurization (ms)"() -> (w278:u32)
                                n186 = Enqueue Element(queue=w275, element=w276, error in (no error)=w274) -> (error out=w273:errorcluster)  [unwired: 1 in, 2 out]
                                n187 = Wait (ms)(milliseconds to wait=w278) -> ()  [unwired: 1 out]
                                }
                                frame "Stop" {
                                w285 = u8[] [0, 0, 0, 0, 0, 11, 0, 16, 0, 0, 0, 2, 4, 255, 0, 0, 0] ("element")
                                n188 = call "Save_current_command.vi"("Array"=w285) -> ()  [unwired: 15 in]
                                n189 = local write "Inlets Flow On"(bool[] [FALSE] ("Inlets On")) -> ()
                                n190 = Byte Array To String(unsigned byte array=w285) -> (string=w289:string)
                                n191 = local read "Start time"() -> (w283:timestamp)
                                n192 = Get Date/Time In Seconds() -> (seconds since 1Jan1904=w284:timestamp)
                                n193 = Subtract(x=w284, y=w283) -> (x-y=w280:dbl)
                                n194 = Divide(x=w280, y=60.0) -> (x/y=→"Elapsed time (min)":dbl)
                                n195 = Enqueue Element(queue=w288, element=w289, error in (no error)=w287) -> (error out=w286:errorcluster)  [unwired: 1 in, 2 out]
                                }
                                }
                                }
                                n196 = Increment(x=w220) -> (x+1=w219:dbl)
                                "Horizontal Graduated Bar" <- w219
                                "Plugs produced" <- w219
                                n197 = local read "Abort"() -> (w228:bool)
                                }
                                n198 = local read "Abort"() -> (w217:bool)
                                n199 = Select(t=T1."Stop", s=w217, f=T1."Barcoding") -> (s? t:f=w218:T1)
                              }
                              frame "Barcoding" {
                                w293 = u8[] [0, 0, 0, 0, 0, 11, 0, 16, 0, 0, 0, 2, 4, 255, 0, 0, 0] ("element")
                                n200 = call "Save_current_command.vi"("Array"=w293) -> ()  [unwired: 15 in]
                                n201 = Byte Array To String(unsigned byte array=w293) -> (string=w297:string)
                                n202 = Enqueue Element(queue=w296, element=w297, error in (no error)=w295) -> (error out=w294:errorcluster)  [unwired: 1 in, 2 out]
                                n203 = local read "Time of barcoding (ms)"() -> (w298:u32)
                                n204 = Wait (ms)(milliseconds to wait=w298) -> ()  [unwired: 1 out]
                              }
                              frame "Stop" {
                                w300 = u8[] [0, 0, 0, 0, 0, 11, 0, 16, 0, 0, 0, 2, 4, 255, 0, 0, 0] ("element")
                                n205 = call "Save_current_command.vi"("Array"=w300) -> ()  [unwired: 15 in]
                                n206 = local write "Inlets Flow On"(bool[] [FALSE] ("Inlets On")) -> ()
                                n207 = Byte Array To String(unsigned byte array=w300) -> (string=w305:string)
                                n208 = Enqueue Element(queue=w303, element=w305, error in (no error)=w302) -> (error out=w301:errorcluster)  [unwired: 1 in, 2 out]
                              }
                            }
                          }
                          n209 = local read "Abort"() -> (w189:bool)
                        }
                      }
                    }
                    frame "Stop" {
                      w329 = TRUE
                      w338 = FALSE
                      # "5"
                      # "4"
                      # "3"
                      # "2"
                      # "1"
                      n210 = local write "Inlet 12"(w338) -> ()
                      n211 = local write "Inlet 13"(w338) -> ()
                      n212 = local write "Inlet 14"(w338) -> ()
                      n213 = local write "Inlet 15"(w338) -> ()
                      n214 = local write "Inlet 16"(w338) -> ()
                      n215 = local write "Inlet 9"(w338) -> ()
                      n216 = local write "Inlet 10"(w338) -> ()
                      n217 = local write "Inlet 11"(w338) -> ()
                      n218 = local write "10"(w329) -> ()
                      n219 = local write "11"(w329) -> ()
                      n220 = local write "12"(w329) -> ()
                      n221 = local write "13"(w329) -> ()
                      n222 = local write "14"(w329) -> ()
                      n223 = local write "15"(w329) -> ()
                      n224 = local write "16"(w329) -> ()
                      n225 = local write "9"(w329) -> ()
                      n226 = local read "10"() -> (w327:bool)
                      n227 = local read "11"() -> (w322:bool)
                      n228 = local read "12"() -> (w321:bool)
                      n229 = local read "13"() -> (w323:bool)
                      n230 = local read "14"() -> (w324:bool)
                      n231 = local read "15"() -> (w325:bool)
                      n232 = local read "16"() -> (w326:bool)
                      n233 = local read "9"() -> (w328:bool)
                      n234 = local write "Plugs produced"(0.0 ("plugs")) -> ()
                      n235 = local read "Start time"() -> (w310:timestamp)
                      n236 = Build Array(w328, w327, w322, w321, w323, w324, w325, w326) -> (w320:bool[])
                      n237 = Get Date/Time In Seconds() -> (seconds since 1Jan1904=w309:timestamp)
                      n238 = local write "Run experiment Button"(FALSE) -> ()
                      n239 = Boolean Array To Number(Boolean array=w320) -> (number=w334:u32)
                      n240 = Subtract(x=w309, y=w310) -> (x-y=w312:dbl)
                      n241 = To Unsigned Byte Integer(number=w334) -> (unsigned 8bit integer=w332:u8)
                      n242 = Divide(x=w312, y=60.0) -> (x/y=w308:dbl)
                      n243 = Build Array (concatenate)(u8[] [0, 0, 0, 0, 0, 11, 0, 16, 0, 0, 0, 2, 4] ("element"), w332, u8[] [0, 0, 0] ("element")) -> (w314:u8[])
                      n244 = local write "Elapsed time (min)"(w308) -> ()
                      n245 = call "Save_current_command.vi"("Array"=w314) -> ()  [unwired: 15 in]
                      n246 = local write "Horizontal Graduated Bar"(u8 0 ("Horizontal Graduated Bar")) -> ()
                      n247 = Byte Array To String(unsigned byte array=w314) -> (string=w333:string)
                      n248 = Enqueue Element(queue=w319, element=w333, error in (no error)=w318) -> (error out=w317:errorcluster)  [unwired: 1 in, 2 out]
                      "Experiment running Led" <- FALSE ("Boolean")
                    }
                  }
                }
              }
            }
          }
        }
        n249 = local read "Stop button"() -> (w85:bool)
      }
      n250 = while {
        tunnel: w12 -> [w353]
        tunnel: w11 -> [w352]
        tunnel: [w349] -> w19
        stop <- w351 stop-if-true
        n251 = event shown="[1] \"9\", \"10\", \"11\", \"12\", \"13\", \"14\", \"15\", \"16\": Value Change" {
          selector: _ -> [_ _ _ _]
          dyn-events: _ -> [_ _ _ _]
          timeout: -1 -> [_ _ _ _]
          tunnel: w352 -> [_ w365 w374 w393]
          tunnel: w353 -> [_ w364 w375 w394]
          tunnel: [_ w355 w373 w392] -> w349
          event Timeout {
            n252 = event-data() -> ()  [unwired: 1 in, 3 out]
          }
          event "9", "10", "11", "12", "13", "14", "15", "16": Value Change {
            # "EVENT 1"
            # "Used for the manual state selection of solenoid valves\nTimeout Value: set to -1 (never to time out)\nInitialisation event: change of value in any of the valve switches (9-16)\n8 control channels -> 8 valves -> 8 switches -> 8 values -> 1 byte"
            n253 = event-data() -> ()  [unwired: 1 in, 6 out]
            n254 = local read "9"() -> (w363:bool)
            n255 = local read "13"() -> (w359:bool)
            n256 = local read "10"() -> (w362:bool)
            n257 = local read "14"() -> (w358:bool)
            n258 = local read "11"() -> (w361:bool)
            n259 = local read "12"() -> (w360:bool)
            n260 = local read "15"() -> (w357:bool)
            n261 = local read "16"() -> (w356:bool)
            n262 = Build Array(w363, w362, w361, w360, w359, w358, w357, w356) -> (w371:bool[])
            n263 = Boolean Array To Number(Boolean array=w371) -> (number=w369:u32)
            n264 = To Unsigned Byte Integer(number=w369) -> (unsigned 8bit integer=w368:u8)
            n265 = Build Array (concatenate)(u8[] [0, 0, 0, 0, 0, 11, 0, 16, 0, 0, 0, 2, 4] ("element"), w368, u8[] [0, 0, 0] ("element")) -> (w354:u8[])
            n266 = call "Save_current_command.vi"("Array"=w354) -> ()  [unwired: 15 in]
            n267 = Byte Array To String(unsigned byte array=w354) -> (string=w366:string)
            n268 = Enqueue Element(queue=w364, element=w366, error in (no error)=w365) -> (error out=w355:errorcluster)  [unwired: 1 in, 2 out]
          }
          event "Depressurize all channels": Value Change {
            w380 = FALSE
            n269 = event-data() -> ()  [unwired: 1 in, 6 out]
            n270 = local write "9"(w380) -> ()
            n271 = local write "10"(w380) -> ()
            n272 = local write "11"(w380) -> ()
            n273 = local write "12"(w380) -> ()
            n274 = local write "13"(w380) -> ()
            n275 = local write "14"(w380) -> ()
            n276 = local write "15"(w380) -> ()
            n277 = local write "16"(w380) -> ()
            n278 = local read "10"() -> (w382:bool)
            n279 = local read "11"() -> (w383:bool)
            n280 = local read "12"() -> (w384:bool)
            n281 = local read "13"() -> (w385:bool)
            n282 = local read "14"() -> (w386:bool)
            n283 = local read "15"() -> (w387:bool)
            n284 = local read "16"() -> (w388:bool)
            n285 = local read "9"() -> (w381:bool)
            n286 = Build Array(w381, w382, w383, w384, w385, w386, w387, w388) -> (w389:bool[])
            n287 = Boolean Array To Number(Boolean array=w389) -> (number=w390:u32)
            n288 = To Unsigned Byte Integer(number=w390) -> (unsigned 8bit integer=w378:u8)
            n289 = Build Array (concatenate)(u8[] [0, 0, 0, 0, 0, 11, 0, 16, 0, 0, 0, 2, 4] ("element"), w378, u8[] [0, 0, 0] ("element")) -> (w372:u8[])
            n290 = call "Save_current_command.vi"("Array"=w372) -> ()  [unwired: 15 in]
            n291 = Byte Array To String(unsigned byte array=w372) -> (string=w379:string)
            n292 = Enqueue Element(queue=w375, element=w379, error in (no error)=w374) -> (error out=w373:errorcluster)  [unwired: 1 in, 2 out]
          }
          event "Pressurize all channels": Value Change {
            w404 = TRUE
            n293 = event-data() -> ()  [unwired: 1 in, 6 out]
            n294 = local write "10"(w404) -> ()
            n295 = local write "11"(w404) -> ()
            n296 = local write "12"(w404) -> ()
            n297 = local write "13"(w404) -> ()
            n298 = local write "14"(w404) -> ()
            n299 = local write "15"(w404) -> ()
            n300 = local write "16"(w404) -> ()
            n301 = local write "9"(w404) -> ()
            n302 = local read "10"() -> (w402:bool)
            n303 = local read "11"() -> (w397:bool)
            n304 = local read "12"() -> (w396:bool)
            n305 = local read "13"() -> (w398:bool)
            n306 = local read "14"() -> (w399:bool)
            n307 = local read "15"() -> (w400:bool)
            n308 = local read "16"() -> (w401:bool)
            n309 = local read "9"() -> (w403:bool)
            n310 = Build Array(w403, w402, w397, w396, w398, w399, w400, w401) -> (w395:bool[])
            n311 = Boolean Array To Number(Boolean array=w395) -> (number=w409:u32)
            n312 = To Unsigned Byte Integer(number=w409) -> (unsigned 8bit integer=w407:u8)
            n313 = Build Array (concatenate)(u8[] [0, 0, 0, 0, 0, 11, 0, 16, 0, 0, 0, 2, 4] ("element"), w407, u8[] [0, 0, 0] ("element")) -> (w391:u8[])
            n314 = call "Save_current_command.vi"("Array"=w391) -> ()  [unwired: 15 in]
            n315 = Byte Array To String(unsigned byte array=w391) -> (string=w408:string)
            n316 = Enqueue Element(queue=w394, element=w408, error in (no error)=w393) -> (error out=w392:errorcluster)  [unwired: 1 in, 2 out]
          }
        }
        n317 = local read "Stop button"() -> (w351:bool)
      }
      n318 = Merge Errors(w21, w20, w19, w14, w10) -> (w27:errorcluster)
      n319 = Release Queue(queue=w15, error in (no error)=w27) -> ()  [unwired: 1 in, 3 out]
    }
  }
